vi "CFG_DataqParams.vi"(11 "Confg File":string[][](array[string])=[["Columns from colC", "12", "Rows From row3", "39", "", "", "", "", "", "", "", "", "", ""], ["", "", "0", "1", "2", "3", "4", "5", "6", "7", "8", "9", "10", "11"], ["Relative Root Name", "PWC-OLS", "Aohm Lo", "Aohm Hi", "A Fill Lo", "A Fill Hi", "A Drain Lo", "A Drain Hi", "Bohm Lo", "Bohm Hi", "B Fill Lo", "B Fill Hi", "B Drain Lo", "B Drain Hi"], ["Test Type", "OLS001", "98", "102", "8.5", "8.5", "8.5", "8.5", "98", "102", "8.5", "8.5", "8.5", "8.5"], ["Resistor Tolerence", "0.01", "98", "102", "7.91", "8.01", "7.55", "7.65", "98", "102", "7.685", "7.785", "7.325", "7.425"], ["Sample Rate", "0.05", "197", "203", "7.46", "7.56", "7.1", "7.2", "197", "203", "7.235", "7.335", "6.875", "6.975"], ["Resistor", "100", "296", "304", "7.01", "7.11", "6.65", "6.75", "296", "304", "6.785", "6.885", "6.425", "6.525"], ["Wait time", "3", "395", "405", "6.56", "6.66", "6.2", "6.3", "395", "405", "6.335", "6.435", "5.975", "6.075"], ["B Level cal", "0", "494", "506", "6.11", "6.21", "5.75", "5.85", "494", "506", "5.885", "5.985", "5.525", "5.625"], ["Sim Fill Rate", "0.002", "593", "607", "5.66", "5.76", "5.3", "5.4", "593", "607", "5.435", "5.535", "5.075", "5.175"], ["Empty Level", "8.4", "692", "708", "5.21", "5.31", "4.85", "4.95", "692", "708", "4.985", "5.085", "4.625", "4.725"], ["Full Level", "2.6", "791", "809", "4.76", "4.86", "4.4", "4.5", "791", "809", "4.535", "4.635", "4.175", "4.275"], ["RNG_Slow", "0.5", "890", "910", "4.31", "4.41", "3.95", "4.05", "890", "910", "4.085", "4.185", "3.725", "3.825"], ["RNG_Creep", "0.007", "989", "1011", "3.86", "3.96", "3.5", "3.6", "989", "1011", "3.635", "3.735", "3.275", "3.375"], ["RNG_Stop", "0.002", "1088", "1112", "3.41", "3.51", "3.05", "3.15", "1088", "1112", "3.185", "3.285", "2.825", "2.925"], ["Laser Slope", "-0.996", "1088", "1112", "2.5", "2.5", "2.5", "2.5", "1088", "1112", "2.5", "2.5", "2.5", "2.5"], ["Laser_Offset", "9.601", "", "", "", "", "", "", "", "", "", "", "", ""], ["Pump Visa Name", "COM4", "", "", "", "", "", "", "", "", "", "", "", ""], ["Zero Settle sec", "5", "", "", "", "", "", "", "", "", "", "", "", ""], ["SPD_Fast", "100", "", "", "", "", "", "", "", "", "", "", "", ""], ["SPD_Slow", "30", "", "", "", "", "", "", "", "", "", "", "", ""], ["SPD_Creep", "7", "", "", "", "", "", "", "", "", "", "", "", ""], ["Level Cal File", "CAL_Level_RnR_241105.xlsx", "", "", "", "", "", "", "", "", "", "", "", ""], ["DataQ Visa Name", "COM3", "", "", "", "", "", "", "", "", "", "", "", ""], ["AI0_Slope", "175.33", "", "", "", "", "", "", "", "", "", "", "", ""], ["AI0_Offset", "2.65678", "", "", "", "", "", "", "", "", "", "", "", ""], ["AI1_Slope", "174.448", "", "", "", "", "", "", "", "", "", "", "", ""], ["AI1_Offset", "3.00272", "", "", "", "", "", "", "", "", "", "", "", ""], ["AI2_Slope", "175", "", "", "", "", "", "", "", "", "", "", "", ""], ["AI2_Offset", "3", "", "", "", "", "", "", "", "", "", "", "", ""], ["AI3_Slope", "175", "", "", "", "", "", "", "", "", "", "", "", ""], ["AI3_Offset", "3", "", "", "", "", "", "", "", "", "", "", "", ""], ["AI4_Slope", "175", "", "", "", "", "", "", "", "", "", "", "", ""], ["AI4_Offset", "3", "", "", "", "", "", "", "", "", "", "", "", ""], ["AI5_Slope", "175", "", "", "", "", "", "", "", "", "", "", "", ""], ["AI5_Offset", "3", "", "", "", "", "", "", "", "", "", "", "", ""], ["AI6_Slope", "175", "", "", "", "", "", "", "", "", "", "", "", ""], ["AI6_Offset", "3", "", "", "", "", "", "", "", "", "", "", "", ""], ["AI7_Slope", "175", "", "", "", "", "", "", "", "", "", "", "", ""], ["AI7_Offset", "3", "", "", "", "", "", "", "", "", "", "", "", ""], ["Report Template", "PWC-OLS\\$ReportFiles\\ReportTemplate_03.xlsx", "", "", "", "", "", "", "", "", "", "", "", ""]]) -> (3 "output cluster":T1={"Visa Name"="", "Num Chan"=0, "Cal Coef"=[], "Scale "=2, "Cal Date"="", "Cal Technicain"=""})   [LabVIEW 2024]
uses:
  DEF_DataqParams.ctl
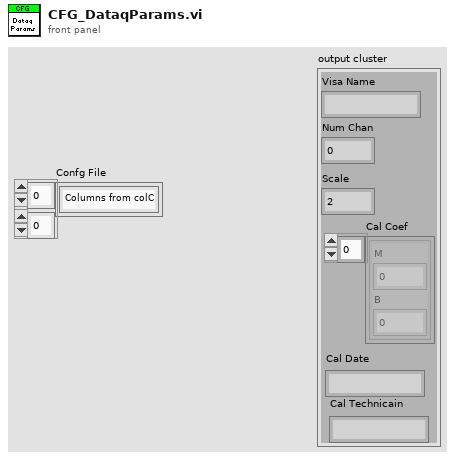
[diagram p1: front panel]
types:
  T1 = typedef "DEF_DataqParams.ctl" = cluster{"Visa Name":string, "Num Chan":i32, "Cal Coef":cluster{"M":dbl, "B":dbl}[], "Scale ":i32, "Cal Date":string, "Cal Technicain":string}
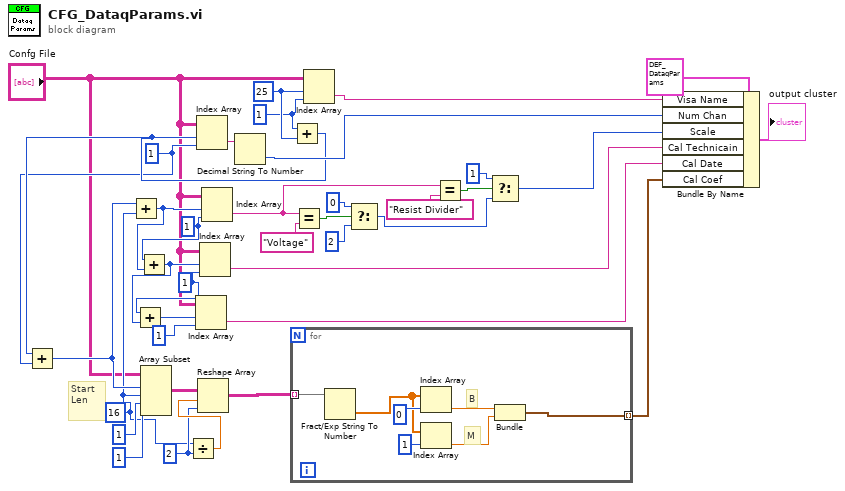
[diagram p0: block diagram]
diagram:
  w14 = 1 ("disabled index (col)")
  w19 = 1 ("disabled index (col)")
  w23 = 1 ("disabled index (col)")
  w32 = 2 ("y")
  w25 = 1 ("disabled index (col)")
  w26 = 25 ("index")
  w21 = 16 ("index")
  # "Start\nLen"
  n1 = Divide(x=w21, y=w32) -> (x/y=w33:dbl)
  n2 = Add(x=w25, y=w26) -> (x+y=w24:i32)
  n3 = Add(x=w24, y=w23) -> (x+y=w22:i32)
  n4 = Add(x=w22, y=w21) -> (x+y=w18:i32)
  n5 = Add(x=w19, y=w18) -> (x+y=w13:i32)
  n6 = Add(x=w14, y=w13) -> (x+y=w15:i32)
  n7 = Array Subset(array="Confg File", index (row)=w22, length (row)=w21, index (col)=1 ("index"), length (col)=1 ("index")) -> (w37:string[][])
  n8 = Index Array(array="Confg File", index (row)=w15, index (col)=1 ("disabled index (col)")) -> (element=w11:string)
  n9 = Index Array(array="Confg File", index (row)=w24, index (col)=w23) -> (element=w30:string)
  n10 = Reshape Array(w37, w33, w32) -> (w31:string[][])
  n11 = Index Array(array="Confg File", index (row)=w13, index (col)=w14) -> (element=w17:string)
  n12 = Index Array(array="Confg File", index (row)=w18, index (col)=w19) -> (element=w4:string)
  n13 = Decimal String To Number(string=w30) -> (number=w27:i32)  [unwired: 2 in, 1 out]
  n14 = for {
    tunnel: w31 -> [w42] mode=indexing
    tunnel: [w38] -> w20 mode=indexing
    # "M"
    # "B"
    n15 = Fract/Exp String To Number(string=w42) -> (number=w41:dbl[])  [unwired: 3 in, 1 out]
    n16 = Index Array(array=w41, index=0) -> (element=w40:dbl)
    n17 = Index Array(array=w41, index=1) -> (element=w39:dbl)
    n18 = Bundle("String"=w40, "String"=w39) -> (w38:cluster{"String":dbl, "String":dbl})  [unwired: 1 in]
  }
  n19 = Equal?(x=w4, y="Voltage") -> (x = y?=w10:bool)
  n20 = Index Array(array="Confg File", index (row)=w26, index (col)=w25) -> (element=w34:string)
  n21 = Select(t=0 ("Scale"), s=w10, f=2 ("Scale")) -> (s? t:f=w3:i32)
  n22 = Equal?(x=w4, y="Resist Divider") -> (x = y?=w8:bool)
  n23 = Select(t=1 ("Scale"), s=w8, f=w3) -> (s? t:f=w1:i32)
  n24 = Bundle By Name(cluster=T1 {"Visa Name"="CAL_Level_RnR_241105.xlsx", "Num Chan"=0, "Cal Coef"=[{"M"=175.33, "B"=2.0}, {"M"=174.448, "B"=2.65678}, {"M"=175.0, "B"=3.00272}, {"M"=175.0, "B"=3.0}, {"M"=175.0, "B"=3.0}, {"M"=175.0, "B"=3.0}, {"M"=175.0, "B"=3.0}, {"M"=175.0, "B"=3.0}], "Scale "=2, "Cal Date"="", "Cal Technicain"=""} ("output cluster"), "Visa Name"=w34, "Num Chan"=w27, "Scale"=w1, "Cal Technicain"=w17, "Cal Date"=w11, "Cal Coef"=w20) -> (→"output cluster":T1)
